vi "Untitled 2.vi"() -> ()   [LabVIEW 2016]
panel:
  out "Array 2":i32[](array[numeric])
  out "Array":i32[](array[numeric])
  out "floor(x/y)":i32
  out "x-y*floor(x/y)":i32
  out "Numeric":i32
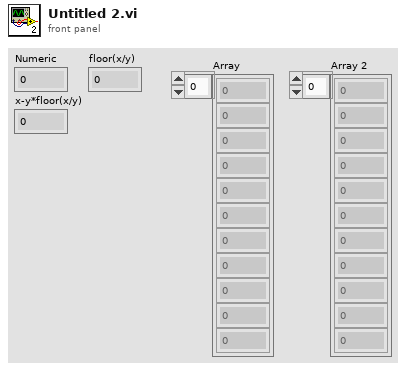
[diagram p1: front panel]
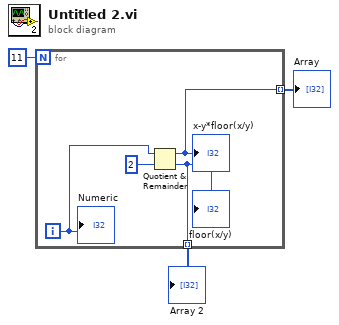
[diagram p0: block diagram]
diagram:
  n1 = for {
    N: 11 -> [_]
    tunnel: [w5] -> w2 mode=indexing
    tunnel: [w4] -> w1 mode=indexing
    i -> [w7]
    n2 = Quotient & Remainder(x=w7, y=2) -> (x-y*floor(x/y)=w5:i32, floor(x/y)=w4:i32)
    "x-y*floor(x/y)" <- w5
    "floor(x/y)" <- w4
    "Numeric" <- w7
  }
  "Array" <- w2
  "Array 2" <- w1
